vi "HFRR ADV v018 new software.vi"() -> ()   [LabVIEW 2025] (continued)
          tunnel: w2021 -> [_ w2088 _ _]
          frame #0 {
            w2037 = "  " ("String 6")
            n2014 = local write "OPEN"(FALSE ("open")) -> ()
            n2015 = local read "string1 2"() -> (w2025:string)
            n2016 = local read "string1 3"() -> (w2024:string)
            n2017 = local read "string1 4"() -> (w2023:string)
            n2018 = property on="OPEN" class="Bool (strict)"("Visible"=FALSE) -> ()  [unwired: 2 in, 2 out]
            n2019 = local write "String 6"(w2037) -> ()
            n2020 = local write "String 7"(w2037) -> ()
            n2021 = local write "String 8"(w2037) -> ()
            n2022 = local write "String 12"(w2037) -> ()
            n2023 = local read "OK Button 16"() -> (w2022:bool)
            n2024 = String To Path(string=w2025) -> (path=w2033:path)
            n2025 = String To Path(string=w2024) -> (path=w2032:path)
            n2026 = String To Path(string=w2023) -> (path=w2031:path)
            n2027 = case shown="True" w2022 {
              tunnel: [w2038 w2039] -> w2026
              frame False {
                n2028 = local read "string1"() -> (w2038:string)
              }
              frame True {
                n2029 = local read "String Indicator 4"() -> (w2039:string)
              }
            }
            n2030 = Open/Create/Replace File "Open File"(file path (use dialog)=w2033) -> (refnum out=w2029:refnum<file>)  [unwired: 5 in, 2 out]
            n2031 = Open/Create/Replace File "Open File"(file path (use dialog)=w2032) -> (refnum out=w2028:refnum<file>)  [unwired: 5 in, 2 out]
            n2032 = Open/Create/Replace File "Open File"(file path (use dialog)=w2031) -> (refnum out=w2027:refnum<file>)  [unwired: 5 in, 2 out]
            n2033 = while {
              tunnel: w2029 -> [w2051]
              i -> [w2047]
              stop <- w2046 continue-if-true
              (unwired) TRUE ("line mode (F)")
              n2034 = Read from Text File "Read File"(file (use dialog)=w2051) -> (text=w2048:string)  [unwired: 3 in, 3 out]
              n2035 = local write "Numeric 11"(w2047) -> ()
              n2036 = String Length(string=w2048) -> (length=w2050:i32)
              n2037 = Greater?(x=w2050, y=1) -> (0:w2046:bool)
            }
            n2038 = while {
              tunnel: w2028 -> [w2057]
              i -> [w2053]
              stop <- w2052 continue-if-true
              (unwired) TRUE ("line mode (F)")
              n2039 = Read from Text File "Read File"(file (use dialog)=w2057) -> (text=w2054:string)  [unwired: 3 in, 3 out]
              n2040 = local write "Numeric 12"(w2053) -> ()
              n2041 = String Length(string=w2054) -> (length=w2056:i32)
              n2042 = Greater?(x=w2056, y=1) -> (0:w2052:bool)
            }
            n2043 = while {
              tunnel: w2027 -> [w2063]
              i -> [w2059]
              stop <- w2058 continue-if-true
              (unwired) TRUE ("line mode (F)")
              n2044 = Read from Text File "Read File"(file (use dialog)=w2063) -> (text=w2060:string)  [unwired: 3 in, 3 out]
              n2045 = local write "Numeric 13"(w2059) -> ()
              n2046 = String Length(string=w2060) -> (length=w2062:i32)
              n2047 = Greater?(x=w2062, y=1) -> (0:w2058:bool)
            }
            n2048 = String To Path(string=w2026) -> (path=w2034:path)
            n2049 = Open/Create/Replace File "Open File"(file path (use dialog)=w2034) -> (refnum out=w2030:refnum<file>)  [unwired: 5 in, 2 out]
            n2050 = while {
              tunnel: w2030 -> [w2045]
              i -> [w2041]
              stop <- w2040 continue-if-true
              (unwired) TRUE ("line mode (F)")
              n2051 = Read from Text File "Read File"(file (use dialog)=w2045) -> (text=w2042:string)  [unwired: 3 in, 3 out]
              n2052 = local write "Numeric 8"(w2041) -> ()
              n2053 = String Length(string=w2042) -> (length=w2044:i32)
              n2054 = Greater?(x=w2044, y=1) -> (0:w2040:bool)
            }
          }
          frame #1 {
            w2215 = FALSE ("ACTUAL   MERGE")
            # "Sample Temp"
            # "ECR"
            # "COF"
            # "Time\nCOF\nFF\nTemp"
            n2055 = case shown="True" w2088 {
              tunnel: [w2235 w2236] -> w2089
              frame False {
                n2056 = local read "string1"() -> (w2235:string)
              }
              frame True {
                n2057 = local read "String Indicator 4"() -> (w2236:string)
              }
            }
            n2058 = local read "string1 3"() -> (w2133:string)
            n2059 = String To Path(string=w2089) -> (path=w2220:path)
            n2060 = String To Path(string=w2133) -> (path=w2231:path)
            n2061 = local read "Numeric 12"() -> (w2217:i32)
            n2062 = local read "Numeric 8"() -> (w2219:i32)
            n2063 = local read "string1 2"() -> (w2134:string)
            n2064 = local read "string1 4"() -> (w2132:string)
            n2065 = Open/Create/Replace File "Open File"(file path (use dialog)=w2220) -> (refnum out=w2234:refnum<file>, error out=w2233:errorcluster)  [unwired: 5 in, 1 out]
            n2066 = Open/Create/Replace File "Open File"(file path (use dialog)=w2231) -> (refnum out=w2227:refnum<file>, error out=w2228:errorcluster)  [unwired: 5 in, 1 out]
            n2067 = for {
              N: w2219 -> [_]
              tunnel: w2234 -> [w2382]
              tunnel: w2233 -> [w2381]
              tunnel: [w2371] -> w2146 mode=indexing
              tunnel: [w2369] -> w2203 mode=indexing
              tunnel: [w2370] -> w2198 mode=indexing
              tunnel: w2215 -> [_]
              tunnel: [w2363] -> w2200 mode=indexing
              tunnel: [w2359] -> w2169 mode=indexing
              tunnel: [w2355] -> w2144 mode=indexing
              tunnel: [w2351] -> w2125 mode=indexing
              tunnel: [w2346] -> w2085 mode=indexing
              (unwired) TRUE ("line mode (F)")
              # "freq"
              # "Stroke"
              # "Time"
              # "CoF"
              # "Humidity"
              # "Temp"
              # "Air Temp"
              # "ECR"
              n2068 = Read from Text File "Read File"(file (use dialog)=w2382, error in=w2381) -> (text=w2347:string)  [unwired: 2 in, 3 out]
              n2069 = local write "String 6"(w2347) -> ()
              n2070 = String Subset(string=w2347, offset (0)=0, length (rest)=14 ("length (rest)")) -> (substring=w2375:string)
              n2071 = String Subset(string=w2347, offset (0)=35, length (rest)=9 ("length (rest)")) -> (substring=w2372:string)
              n2072 = String Subset(string=w2347, offset (0)=15, length (rest)=9 ("length (rest)")) -> (substring=w2378:string)
              n2073 = Fract/Exp String To Number(string=w2375) -> (number=w2371:dbl)  [unwired: 3 in, 1 out]
              n2074 = Fract/Exp String To Number(string=w2372) -> (number=w2370:dbl)  [unwired: 3 in, 1 out]
              n2075 = Fract/Exp String To Number(string=w2378) -> (number=w2369:dbl)  [unwired: 3 in, 1 out]
              n2076 = String Subset(string=w2347, offset (0)=85, length (rest)=9 ("length (rest)")) -> (substring=w2348:string)
              n2077 = String Subset(string=w2347, offset (0)=25, length (rest)=9 ("length (rest)")) -> (substring=w2354:string)
              n2078 = String Subset(string=w2347, offset (0)=55, length (rest)=9 ("length (rest)")) -> (substring=w2356:string)
              n2079 = String Subset(string=w2347, offset (0)=45, length (rest)=9 ("length (rest)")) -> (substring=w2362:string)
              n2080 = String Subset(string=w2347, offset (0)=65, length (rest)=9 ("length (rest)")) -> (substring=w2368:string)
              n2081 = Fract/Exp String To Number(string=w2354) -> (number=w2351:dbl)  [unwired: 3 in, 1 out]
              n2082 = Fract/Exp String To Number(string=w2348) -> (number=w2346:dbl)  [unwired: 3 in, 1 out]
              n2083 = Fract/Exp String To Number(string=w2356) -> (number=w2355:dbl)  [unwired: 3 in, 1 out]
              n2084 = Fract/Exp String To Number(string=w2362) -> (number=w2359:dbl)  [unwired: 3 in, 1 out]
              n2085 = Fract/Exp String To Number(string=w2368) -> (number=w2365:dbl)  [unwired: 3 in, 1 out]
              n2086 = Add(x=w2365, y=0.0) -> (x+y=w2363:dbl)
            }
            n2087 = for {
              N: w2217 -> [_]
              tunnel: w2228 -> [w2308]
              tunnel: w2227 -> [w2307]
              tunnel: [w2297] -> w2186 mode=indexing
              tunnel: [w2295] -> w2184 mode=indexing
              tunnel: [w2296] -> w2180 mode=indexing
              tunnel: w2215 -> [_]
              tunnel: [w2289] -> w2182 mode=indexing
              tunnel: [w2285] -> w2164 mode=indexing
              tunnel: [w2281] -> w2140 mode=indexing
              tunnel: [w2278] -> w2121 mode=indexing
              tunnel: [w2274] -> w2080 mode=indexing
              (unwired) 9 ("length (rest)")
              (unwired) 9 ("length (rest)")
              (unwired) TRUE ("line mode (F)")
              n2088 = Read from Text File "Read File"(file (use dialog)=w2307, error in=w2308) -> (text=w2275:string)  [unwired: 2 in, 3 out]
              n2089 = local write "String 8"(w2275) -> ()
              n2090 = String Subset(string=w2275, offset (0)=85) -> (substring=w2277:string)  [unwired: 1 in]
              n2091 = String Subset(string=w2275, offset (0)=35, length (rest)=9 ("length (rest)")) -> (substring=w2298:string)
              n2092 = String Subset(string=w2275, offset (0)=55, length (rest)=9 ("length (rest)")) -> (substring=w2283:string)
              n2093 = String Subset(string=w2275, offset (0)=25) -> (substring=w2279:string)  [unwired: 1 in]
              n2094 = String Subset(string=w2275, offset (0)=15, length (rest)=9 ("length (rest)")) -> (substring=w2304:string)
              n2095 = String Subset(string=w2275, offset (0)=0, length (rest)=14 ("length (rest)")) -> (substring=w2301:string)
              n2096 = String Subset(string=w2275, offset (0)=45, length (rest)=9 ("length (rest)")) -> (substring=w2288:string)
              n2097 = String Subset(string=w2275, offset (0)=65, length (rest)=9 ("length (rest)")) -> (substring=w2294:string)
              n2098 = Fract/Exp String To Number(string=w2277) -> (number=w2274:dbl)  [unwired: 3 in, 1 out]
              n2099 = Fract/Exp String To Number(string=w2298) -> (number=w2296:dbl)  [unwired: 3 in, 1 out]
              n2100 = Fract/Exp String To Number(string=w2283) -> (number=w2281:dbl)  [unwired: 3 in, 1 out]
              n2101 = Fract/Exp String To Number(string=w2279) -> (number=w2278:dbl)  [unwired: 3 in, 1 out]
              n2102 = Fract/Exp String To Number(string=w2304) -> (number=w2295:dbl)  [unwired: 3 in, 1 out]
              n2103 = Fract/Exp String To Number(string=w2301) -> (number=w2297:dbl)  [unwired: 3 in, 1 out]
              n2104 = Fract/Exp String To Number(string=w2288) -> (number=w2285:dbl)  [unwired: 3 in, 1 out]
              n2105 = Fract/Exp String To Number(string=w2294) -> (number=w2291:dbl)  [unwired: 3 in, 1 out]
              n2106 = Add(x=w2291, y=0.0) -> (x+y=w2289:dbl)
            }
            n2107 = String To Path(string=w2134) -> (path=w2232:path)
            n2108 = String To Path(string=w2132) -> (path=w2226:path)
            n2109 = local read "Numeric 11"() -> (w2216:i32)
            n2110 = local read "Numeric 13"() -> (w2218:i32)
            n2111 = Open/Create/Replace File "Open File"(file path (use dialog)=w2232) -> (refnum out=w2230:refnum<file>, error out=w2229:errorcluster)  [unwired: 5 in, 1 out]
            n2112 = Open/Create/Replace File "Open File"(file path (use dialog)=w2226) -> (refnum out=w2225:refnum<file>, error out=w2224:errorcluster)  [unwired: 5 in, 1 out]
            n2113 = for {
              N: w2216 -> [_]
              tunnel: w2230 -> [w2345]
              tunnel: w2229 -> [w2344]
              tunnel: [w2334] -> w2196 mode=indexing
              tunnel: [w2332] -> w2194 mode=indexing
              tunnel: [w2333] -> w2189 mode=indexing
              tunnel: w2215 -> [_]
              tunnel: [w2326] -> w2191 mode=indexing
              tunnel: [w2322] -> w2167 mode=indexing
              tunnel: [w2318] -> w2142 mode=indexing
              tunnel: [w2314] -> w2123 mode=indexing
              tunnel: [w2309] -> w2081 mode=indexing
              (unwired) TRUE ("line mode (F)")
              n2114 = Read from Text File "Read File"(file (use dialog)=w2345, error in=w2344) -> (text=w2310:string)  [unwired: 2 in, 3 out]
              n2115 = local write "String 7"(w2310) -> ()
              n2116 = String Subset(string=w2310, offset (0)=85, length (rest)=9 ("length (rest)")) -> (substring=w2313:string)
              n2117 = String Subset(string=w2310, offset (0)=35, length (rest)=9 ("length (rest)")) -> (substring=w2335:string)
              n2118 = String Subset(string=w2310, offset (0)=55, length (rest)=9 ("length (rest)")) -> (substring=w2321:string)
              n2119 = String Subset(string=w2310, offset (0)=25, length (rest)=9 ("length (rest)")) -> (substring=w2315:string)
              n2120 = String Subset(string=w2310, offset (0)=45, length (rest)=9 ("length (rest)")) -> (substring=w2323:string)
              n2121 = String Subset(string=w2310, offset (0)=0, length (rest)=14 ("length (rest)")) -> (substring=w2338:string)
              n2122 = String Subset(string=w2310, offset (0)=15, length (rest)=9 ("length (rest)")) -> (substring=w2341:string)
              n2123 = String Subset(string=w2310, offset (0)=65, length (rest)=9 ("length (rest)")) -> (substring=w2327:string)
              n2124 = Fract/Exp String To Number(string=w2313) -> (number=w2309:dbl)  [unwired: 3 in, 1 out]
              n2125 = Fract/Exp String To Number(string=w2335) -> (number=w2333:dbl)  [unwired: 3 in, 1 out]
              n2126 = Fract/Exp String To Number(string=w2321) -> (number=w2318:dbl)  [unwired: 3 in, 1 out]
              n2127 = Fract/Exp String To Number(string=w2315) -> (number=w2314:dbl)  [unwired: 3 in, 1 out]
              n2128 = Fract/Exp String To Number(string=w2323) -> (number=w2322:dbl)  [unwired: 3 in, 1 out]
              n2129 = Fract/Exp String To Number(string=w2338) -> (number=w2334:dbl)  [unwired: 3 in, 1 out]
              n2130 = Fract/Exp String To Number(string=w2341) -> (number=w2332:dbl)  [unwired: 3 in, 1 out]
              n2131 = Fract/Exp String To Number(string=w2327) -> (number=w2330:dbl)  [unwired: 3 in, 1 out]
              n2132 = Add(x=w2330, y=0.0) -> (x+y=w2326:dbl)
            }
            n2133 = for {
              N: w2218 -> [_]
              tunnel: w2225 -> [w2273]
              tunnel: w2224 -> [w2272]
              tunnel: [w2262] -> w2178 mode=indexing
              tunnel: [w2261] -> w2171 mode=indexing
              tunnel: w2215 -> [_]
              tunnel: [w2250] -> w2176 mode=indexing
              tunnel: [w2255] -> w2173 mode=indexing
              tunnel: [w2251] -> w2163 mode=indexing
              tunnel: [w2246] -> w2138 mode=indexing
              tunnel: [w2242] -> w2119 mode=indexing
              tunnel: [w2237] -> w2079 mode=indexing
              (unwired) 1.0 ("x")
              (unwired) TRUE ("line mode (F)")
              n2134 = Read from Text File "Read File"(file (use dialog)=w2273, error in=w2272) -> (text=w2238:string)  [unwired: 2 in, 3 out]
              n2135 = local write "String 12"(w2238) -> ()
              n2136 = String Subset(string=w2238, offset (0)=85, length (rest)=9 ("length (rest)")) -> (substring=w2240:string)
              n2137 = String Subset(string=w2238, offset (0)=35, length (rest)=9 ("length (rest)")) -> (substring=w2263:string)
              n2138 = String Subset(string=w2238, offset (0)=55, length (rest)=9 ("length (rest)")) -> (substring=w2248:string)
              n2139 = String Subset(string=w2238, offset (0)=25, length (rest)=9 ("length (rest)")) -> (substring=w2244:string)
              n2140 = String Subset(string=w2238, offset (0)=45, length (rest)=9 ("length (rest)")) -> (substring=w2253:string)
              n2141 = String Subset(string=w2238, offset (0)=15, length (rest)=9 ("length (rest)")) -> (substring=w2269:string)
              n2142 = String Subset(string=w2238, offset (0)=0, length (rest)=14 ("length (rest)")) -> (substring=w2266:string)
              n2143 = String Subset(string=w2238, offset (0)=65, length (rest)=9 ("length (rest)")) -> (substring=w2256:string)
              n2144 = Fract/Exp String To Number(string=w2240) -> (number=w2237:dbl)  [unwired: 3 in, 1 out]
              n2145 = Fract/Exp String To Number(string=w2263) -> (number=w2261:dbl)  [unwired: 3 in, 1 out]
              n2146 = Fract/Exp String To Number(string=w2248) -> (number=w2246:dbl)  [unwired: 3 in, 1 out]
              n2147 = Fract/Exp String To Number(string=w2244) -> (number=w2242:dbl)  [unwired: 3 in, 1 out]
              n2148 = Fract/Exp String To Number(string=w2253) -> (number=w2251:dbl)  [unwired: 3 in, 1 out]
              n2149 = Fract/Exp String To Number(string=w2269) -> (number=w2250:dbl)  [unwired: 3 in, 1 out]
              n2150 = Fract/Exp String To Number(string=w2266) -> (number=w2262:dbl)  [unwired: 3 in, 1 out]
              n2151 = Fract/Exp String To Number(string=w2256) -> (number=w2259:dbl)  [unwired: 3 in, 1 out]
              n2152 = Add(x=w2259, y=0.0) -> (x+y=w2255:dbl)
            }
            n2153 = Delete From Array(array=w2121, index=0) -> (array with subset deleted=w2094:dbl[])  [unwired: 1 in, 1 out]
            n2154 = Delete From Array(array=w2184, index=0) -> (array with subset deleted=w2157:dbl[])  [unwired: 1 in, 1 out]
            n2155 = Delete From Array(array=w2164, index=0) -> (array with subset deleted=w2152:dbl[])  [unwired: 1 in, 1 out]
            n2156 = Delete From Array(array=w2182, index=0) -> (array with subset deleted=w2183:dbl[])  [unwired: 1 in, 1 out]
            n2157 = call-poly <vilib>:"Mean.vi"("X"=w2094) -> ("mean"=→"КОФ2 4":dbl)  [unwired: 1 out]
            n2158 = call-poly <vilib>:"Mean.vi"("X"=w2157) -> ("mean"=→"КОФ3":dbl)  [unwired: 1 out]
            n2159 = call-poly <vilib>:"Mean.vi"("X"=w2152) -> ("mean"=→"CP3":dbl)  [unwired: 1 out]
            n2160 = Delete From Array(array=w2146, index=0) -> (array with subset deleted=w2073:dbl[])  [unwired: 1 in, 1 out]
            n2161 = Delete From Array(array=w2085, index=0) -> (array with subset deleted=w2072:dbl[])  [unwired: 1 in, 1 out]
            n2162 = Delete From Array(array=w2125, index=0) -> (array with subset deleted=w2096:dbl[])  [unwired: 1 in, 1 out]
            n2163 = Delete From Array(array=w2203, index=0) -> (array with subset deleted=w2158:dbl[])  [unwired: 1 in, 1 out]
            n2164 = Delete From Array(array=w2169, index=0) -> (array with subset deleted=w2154:dbl[])  [unwired: 1 in, 1 out]
            "array w/ subset deleted" <- w2154
            n2165 = Delete From Array(array=w2200, index=0) -> (array with subset deleted=w2201:dbl[])  [unwired: 1 in, 1 out]
            n2166 = call-poly <vilib>:"Mean.vi"("X"=w2096) -> ("mean"=→"КОФ2 2":dbl)  [unwired: 1 out]
            n2167 = call-poly <vilib>:"Mean.vi"("X"=w2158) -> ("mean"=→"КОФ1":dbl)  [unwired: 1 out]
            n2168 = Bundle "Bundle"(w2073, w2072) -> (w2078:cluster{dbl[], dbl[]})  [unwired: 1 in]
            n2169 = Bundle "Bundle"(w2073, w2201) -> (w2065:cluster{dbl[], dbl[]})  [unwired: 1 in]
            n2170 = Delete From Array(array=w2080, index=0) -> (array with subset deleted=w2068:dbl[])  [unwired: 1 in, 1 out]
            n2171 = Delete From Array(array=w2081, index=0) -> (array with subset deleted=w2070:dbl[])  [unwired: 1 in, 1 out]
            n2172 = Delete From Array(array=w2191, index=0) -> (array with subset deleted=w2192:dbl[])  [unwired: 1 in, 1 out]
            n2173 = Delete From Array(array=w2079, index=0) -> (array with subset deleted=w2066:dbl[])  [unwired: 1 in, 1 out]
            n2174 = Delete From Array(array=w2173, index=0) -> (array with subset deleted=w2174:dbl[])  [unwired: 1 in, 1 out]
            n2175 = Delete From Array(array=w2198, index=0) -> (array with subset deleted=w2104:dbl[])  [unwired: 1 in, 1 out]
            n2176 = Delete From Array(array=w2144, index=0) -> (array with subset deleted=w2100:dbl[])  [unwired: 1 in, 1 out]
            n2177 = Delete From Array(array=w2180, index=0) -> (array with subset deleted=w2102:dbl[])  [unwired: 1 in, 1 out]
            n2178 = Delete From Array(array=w2140, index=0) -> (array with subset deleted=w2098:dbl[])  [unwired: 1 in, 1 out]
            n2179 = Delete From Array(array=w2189, index=0) -> (array with subset deleted=w2103:dbl[])  [unwired: 1 in, 1 out]
            n2180 = Delete From Array(array=w2142, index=0) -> (array with subset deleted=w2099:dbl[])  [unwired: 1 in, 1 out]
            n2181 = Delete From Array(array=w2123, index=0) -> (array with subset deleted=w2095:dbl[])  [unwired: 1 in, 1 out]
            n2182 = Delete From Array(array=w2167, index=0) -> (array with subset deleted=w2153:dbl[])  [unwired: 1 in, 1 out]
            n2183 = Delete From Array(array=w2194, index=0) -> (array with subset deleted=w2155:dbl[])  [unwired: 1 in, 1 out]
            n2184 = Delete From Array(array=w2171, index=0) -> (array with subset deleted=w2101:dbl[])  [unwired: 1 in, 1 out]
            n2185 = Delete From Array(array=w2138, index=0) -> (array with subset deleted=w2097:dbl[])  [unwired: 1 in, 1 out]
            n2186 = Delete From Array(array=w2119, index=0) -> (array with subset deleted=w2093:dbl[])  [unwired: 1 in, 1 out]
            n2187 = Delete From Array(array=w2163, index=0) -> (array with subset deleted=w2151:dbl[])  [unwired: 1 in, 1 out]
            n2188 = Delete From Array(array=w2176, index=0) -> (array with subset deleted=w2156:dbl[])  [unwired: 1 in, 1 out]
            n2189 = Delete From Array(array=w2186, index=0) -> (array with subset deleted=w2069:dbl[])  [unwired: 1 in, 1 out]
            n2190 = Delete From Array(array=w2196, index=0) -> (array with subset deleted=w2071:dbl[])  [unwired: 1 in, 1 out]
            n2191 = Delete From Array(array=w2178, index=0) -> (array with subset deleted=w2067:dbl[])  [unwired: 1 in, 1 out]
            n2192 = Bundle "Bundle"(w2073, w2104) -> (w2091:cluster{dbl[], dbl[]})  [unwired: 1 in]
            n2193 = Bundle "Bundle"(w2073, w2158) -> (w2092:cluster{dbl[], dbl[]})  [unwired: 1 in]
            n2194 = Bundle "Bundle"(w2104, w2100) -> (w2106:cluster{dbl[], dbl[]})  [unwired: 1 in]
            n2195 = Bundle "Bundle"(w2069, w2068) -> (w2076:cluster{dbl[], dbl[]})  [unwired: 1 in]
            n2196 = Bundle "Bundle"(w2102, w2098) -> (w2108:cluster{dbl[], dbl[]})  [unwired: 1 in]
            n2197 = Bundle "Bundle"(w2069, w2102) -> (w2212:cluster{dbl[], dbl[]})  [unwired: 1 in]
            n2198 = Bundle "Bundle"(w2069, w2098) -> (w2136:cluster{dbl[], dbl[]})  [unwired: 1 in]
            n2199 = Bundle "Bundle"(w2069, w2157) -> (w2222:cluster{dbl[], dbl[]})  [unwired: 1 in]
            n2200 = Bundle "Bundle"(w2069, w2152) -> (w2160:cluster{dbl[], dbl[]})  [unwired: 1 in]
            n2201 = Bundle "Bundle"(w2069, w2183) -> (w2207:cluster{dbl[], dbl[]})  [unwired: 1 in]
            n2202 = Bundle "Bundle"(w2103, w2099) -> (w2107:cluster{dbl[], dbl[]})  [unwired: 1 in]
            n2203 = Bundle "Bundle"(w2071, w2070) -> (w2077:cluster{dbl[], dbl[]})  [unwired: 1 in]
            n2204 = Bundle "Bundle"(w2071, w2103) -> (w2214:cluster{dbl[], dbl[]})  [unwired: 1 in]
            n2205 = Bundle "Bundle"(w2071, w2099) -> (w2137:cluster{dbl[], dbl[]})  [unwired: 1 in]
            n2206 = Bundle "Bundle"(w2071, w2153) -> (w2161:cluster{dbl[], dbl[]})  [unwired: 1 in]
            n2207 = Bundle "Bundle"(w2071, w2155) -> (w2223:cluster{dbl[], dbl[]})  [unwired: 1 in]
            n2208 = Bundle "Bundle"(w2071, w2192) -> (w2205:cluster{dbl[], dbl[]})  [unwired: 1 in]
            n2209 = Bundle "Bundle"(w2101, w2097) -> (w2109:cluster{dbl[], dbl[]})  [unwired: 1 in]
            n2210 = Bundle "Bundle"(w2067, w2066) -> (w2075:cluster{dbl[], dbl[]})  [unwired: 1 in]
            n2211 = Bundle "Bundle"(w2067, w2101) -> (w2213:cluster{dbl[], dbl[]})  [unwired: 1 in]
            n2212 = Bundle "Bundle"(w2067, w2097) -> (w2135:cluster{dbl[], dbl[]})  [unwired: 1 in]
            n2213 = Bundle "Bundle"(w2067, w2151) -> (w2159:cluster{dbl[], dbl[]})  [unwired: 1 in]
            n2214 = Bundle "Bundle"(w2067, w2156) -> (w2221:cluster{dbl[], dbl[]})  [unwired: 1 in]
            n2215 = Bundle "Bundle"(w2067, w2174) -> (w2206:cluster{dbl[], dbl[]})  [unwired: 1 in]
            n2216 = call-poly <vilib>:"Mean.vi"("X"=w2154) -> ("mean"=→"CP1":dbl)  [unwired: 1 out]
            n2217 = call-poly <vilib>:"Mean.vi"("X"=w2095) -> ("mean"=→"КОФ2 3":dbl)  [unwired: 1 out]
            n2218 = call-poly <vilib>:"Mean.vi"("X"=w2153) -> ("mean"=→"CP2":dbl)  [unwired: 1 out]
            n2219 = call-poly <vilib>:"Mean.vi"("X"=w2155) -> ("mean"=→"КОФ2":dbl)  [unwired: 1 out]
            n2220 = call-poly <vilib>:"Mean.vi"("X"=w2093) -> ("mean"=→"КОФ2 5":dbl)  [unwired: 1 out]
            n2221 = call-poly <vilib>:"Mean.vi"("X"=w2151) -> ("mean"=→"CP4":dbl)  [unwired: 1 out]
            n2222 = call-poly <vilib>:"Mean.vi"("X"=w2156) -> ("mean"=→"КОФ4":dbl)  [unwired: 1 out]
            n2223 = Bundle "Bundle"(w2073, w2100) -> (w2064:cluster{dbl[], dbl[]})  [unwired: 1 in]
            n2224 = Bundle "Bundle"(w2073, w2154) -> (w2087:cluster{dbl[], dbl[]})  [unwired: 1 in]
            n2225 = Build Array "Build Array"(w2064, w2087) -> (w2090:cluster{dbl[], dbl[]}[])
            "XY Graph 17" <- w2090
            n2226 = Build Array "Build Array"(w2078, w2077, w2076, w2075) -> (→"Frequency ( Hz )":cluster{dbl[], dbl[]}[])
            n2227 = Build Array "Build Array"(w2106, w2107, w2108, w2109) -> (→"Air Temp ( °C ) vs Humidity ( % RH )":cluster{dbl[], dbl[]}[])
            n2228 = Build Array "Build Array"(w2091, w2214, w2212, w2213) -> (→"Air Temperature  ( °C )":cluster{dbl[], dbl[]}[])
            n2229 = Build Array "Build Array"(w2064, w2137, w2136, w2135) -> (→"Humidity ( %RH )":cluster{dbl[], dbl[]}[])
            n2230 = Build Array "Build Array"(w2092, w2223, w2222, w2221) -> (→"Coefficient Of Friction":cluster{dbl[], dbl[]}[])
            n2231 = Build Array "Build Array"(w2087, w2161, w2160, w2159) -> (→"Sample Temperature ( °C )":cluster{dbl[], dbl[]}[])
            n2232 = Build Array "Build Array"(w2065, w2205, w2207, w2206) -> (→"XY Graph 13":cluster{dbl[], dbl[]}[])
            n2233 = Bundle "Bundle"(w2073, w2096) -> (w2118:cluster{dbl[], dbl[]})  [unwired: 1 in]
            n2234 = Bundle "Bundle"(w2069, w2094) -> (w2116:cluster{dbl[], dbl[]})  [unwired: 1 in]
            n2235 = Bundle "Bundle"(w2071, w2095) -> (w2117:cluster{dbl[], dbl[]})  [unwired: 1 in]
            n2236 = Bundle "Bundle"(w2067, w2093) -> (w2115:cluster{dbl[], dbl[]})  [unwired: 1 in]
            n2237 = Build Array "Build Array"(w2118, w2117, w2116, w2115) -> (→"Stroke ( mm )":cluster{dbl[], dbl[]}[])
            n2238 = local write "XY Graph 16"(w2090) -> ()
          }
          frame #2 {
          }
          frame #3 {
            n2239 = local write "Numeric 8"(0 ("Numeric 8")) -> ()
            n2240 = local write "Numeric 11"(0 ("Numeric 11")) -> ()
            n2241 = local write "Numeric 12"(0 ("Numeric 12")) -> ()
            n2242 = local write "Numeric 13"(0 ("Numeric 13")) -> ()
            n2243 = property on="OPEN" class="Bool (strict)"("Visible"=TRUE) -> ()  [unwired: 2 in, 2 out]
            n2244 = local read "String Control 2"() -> (w2390:string)
            n2245 = local read "String Control 4"() -> (w2389:string)
            n2246 = local read "String Control 6"() -> (w2388:string)
            n2247 = local read "String Control 8"() -> (w2387:string)
            n2248 = Match Pattern(string=w2390, regular expression="Samples / cycle :- ") -> (after substring=w2404:string)  [unwired: 1 in, 3 out]
            n2249 = Match Pattern(string=w2390, regular expression="Frequency :- ") -> (after substring=w2423:string)  [unwired: 1 in, 3 out]
            n2250 = Match Pattern(string=w2389, regular expression="Samples / cycle :- ") -> (after substring=w2400:string)  [unwired: 1 in, 3 out]
            n2251 = Match Pattern(string=w2389, regular expression="Frequency :- ") -> (after substring=w2418:string)  [unwired: 1 in, 3 out]
            n2252 = Match Pattern(string=w2388, regular expression="Samples / cycle :- ") -> (after substring=w2396:string)  [unwired: 1 in, 3 out]
            n2253 = Match Pattern(string=w2388, regular expression="Frequency :- ") -> (after substring=w2413:string)  [unwired: 1 in, 3 out]
            n2254 = Match Pattern(string=w2387, regular expression="Samples / cycle :- ") -> (after substring=w2392:string)  [unwired: 1 in, 3 out]
            n2255 = Match Pattern(string=w2387, regular expression="Frequency :- ") -> (after substring=w2408:string)  [unwired: 1 in, 3 out]
            n2256 = String Subset(string=w2404, length (rest)=6 ("length (rest)")) -> (substring=w2406:string)  [unwired: 1 in]
            n2257 = String Subset(string=w2423, length (rest)=9 ("length (rest)")) -> (substring=w2425:string)  [unwired: 1 in]
            n2258 = String Subset(string=w2400, length (rest)=6 ("length (rest)")) -> (substring=w2402:string)  [unwired: 1 in]
            n2259 = String Subset(string=w2418, length (rest)=9 ("length (rest)")) -> (substring=w2420:string)  [unwired: 1 in]
            n2260 = String Subset(string=w2396, length (rest)=6 ("length (rest)")) -> (substring=w2398:string)  [unwired: 1 in]
            n2261 = String Subset(string=w2413, length (rest)=9 ("length (rest)")) -> (substring=w2415:string)  [unwired: 1 in]
            n2262 = String Subset(string=w2392, length (rest)=6 ("length (rest)")) -> (substring=w2394:string)  [unwired: 1 in]
            n2263 = String Subset(string=w2408, length (rest)=9 ("length (rest)")) -> (substring=w2410:string)  [unwired: 1 in]
            n2264 = Fract/Exp String To Number(string=w2406) -> (number=w2386:dbl)  [unwired: 3 in, 1 out]
            n2265 = Fract/Exp String To Number(string=w2425) -> (number=w2426:dbl)  [unwired: 3 in, 1 out]
            n2266 = Fract/Exp String To Number(string=w2402) -> (number=w2385:dbl)  [unwired: 3 in, 1 out]
            n2267 = Fract/Exp String To Number(string=w2420) -> (number=w2421:dbl)  [unwired: 3 in, 1 out]
            n2268 = Fract/Exp String To Number(string=w2398) -> (number=w2384:dbl)  [unwired: 3 in, 1 out]
            n2269 = Fract/Exp String To Number(string=w2415) -> (number=w2416:dbl)  [unwired: 3 in, 1 out]
            n2270 = Fract/Exp String To Number(string=w2394) -> (number=w2383:dbl)  [unwired: 3 in, 1 out]
            n2271 = Fract/Exp String To Number(string=w2410) -> (number=w2411:dbl)  [unwired: 3 in, 1 out]
            n2272 = local write "sample1"(w2386) -> ()
            n2273 = local write "freq1"(w2426) -> ()
            n2274 = local write "sample2"(w2385) -> ()
            n2275 = local write "freq2"(w2421) -> ()
            n2276 = local write "sample3"(w2384) -> ()
            n2277 = local write "freq3"(w2416) -> ()
            n2278 = local write "sample4"(w2383) -> ()
            n2279 = local write "freq 4"(w2411) -> ()
          }
        }
      }
    }
    n2280 = case shown="True" w1875 {
      selector: w1875 -> [_ w2003]
      frame False {
      }
      frame True {
        n2281 = Not(x=w2003) -> (.not. x?=w1999:bool)
        n2282 = local write "service 3"(w1999) -> ()
        n2283 = local write "OPEN 6"(w1999) -> ()
        n2284 = call <vilib>:"System Exec.vi"("wait until completion? (T)"=TRUE, "command line"="C:\\LAB-IQ\\Scar View.exe") -> ("error out"=→"error out 5":errorcluster)  [unwired: 6 in, 3 out]
      }
    }
    n2285 = case shown="\"Acquire\", Default" w1886 {
      frame "Acquire", Default {
        w2899 = 0.2 ("y")
        w2904 = 1.0 ("y")
        w2905 = 0.8 ("y")
        # "Elapsed time\ncof\nstroke\nAir temp\nTemp\nHumidity"
        n2286 = disable-structure shown="Disabled" {
          frame Disabled {
            n2287 = local read "Flag"() -> (w2922:dbl)
            n2288 = local read "RUN"() -> (w2919:bool)
            n2289 = Not(x=w2919) -> (.not. x?=w2918:bool)
            n2290 = Equal?(x=w2922, y=10.0) -> (x = y?=w2920:bool)
            n2291 = And(x=w2920, y=w2918) -> (x .and. y?=w2917:bool)
            n2292 = case shown="True" w2917 {
              frame False {
              }
              frame True {
                w2923 = FALSE ("Heater Button")
                n2293 = local write "Humidity"(w2923) -> ()
                n2294 = local write "Heater Button"(w2923) -> ()
              }
            }
          }
          frame Enabled {
          }
        }
        n2295 = disable-structure shown="Disabled" {
          frame Disabled {
            n2296 = case shown="True" {
              selector: _ -> [_ _]
              frame False {
              }
              frame True {
                w3014 = TRUE ("Heater")
                n2297 = local write "Humidity"(w3014) -> ()
                n2298 = local write "Heater Button"(w3014) -> ()
                n2299 = local read "TEST STANDARD"() -> (w3017:T3)
                n2300 = local read "TEST STANDARD"() -> (w3012:T3)
                n2301 = Equal?(x=w3017, y=enum16{"ASTM D6079", "ISO 12156", "Custom"}."ISO 12156" ("Test Standard")) -> (x = y?=w3015:bool)
                n2302 = Equal?(x=w3012, y=enum16{"ASTM D6079", "ISO 12156", "Custom"}."ASTM D6079" ("Test Standard")) -> (x = y?=w3011:bool)
                n2303 = case shown="True" w3015 {
                  frame False {
                  }
                  frame True {
                    n2304 = local write "Heater"(TRUE ("Heater")) -> ()
                    n2305 = local write "airtempflg"(FALSE ("airtempflg")) -> ()
                  }
                }
                n2306 = case shown="True" w3011 {
                  frame False {
                  }
                  frame True {
                    n2307 = local write "Heater"(FALSE ("Heater")) -> ()
                    n2308 = local write "airtempflg"(TRUE ("airtempflg")) -> ()
                  }
                }
              }
            }
          }
          frame Enabled {
          }
        }
        n2309 = stacked-sequence {
          frame #0 {
            n2310 = case shown="True" "RST FF" {
              frame False {
              }
              frame True {
                w3080 = 0.0 ("X Scale.Range:Maximum")
                n2311 = property on="Frictional Force ( N )" class="WFChart (strict)"("XScale.Maximum"=600.0 ("X Scale.Range:Maximum"), "XScale.Minimum"=w3080, "YScale.Maximum"=10.0 ("Y Scale.Range:Maximum"), "YScale.Minimum"=w3080) -> ()  [unwired: 2 in, 2 out]
              }
            }
          }
          frame #1 {
            n2312 = case shown="True" "RST TEMP" {
              frame False {
              }
              frame True {
                n2313 = property on="Temperature ( Deg C )" class="WFChart (strict)"("XScale.Minimum"=0.0 ("X Scale.Range:Minimum"), "XScale.Maximum"=600.0 ("X Scale.Range:Maximum"), "YScale.Minimum"=0.0 ("Y Scale.Range:Minimum"), "YScale.Maximum"=100.0 ("Y Scale.Range:Maximum")) -> ()  [unwired: 2 in, 2 out]
              }
            }
          }
          frame #2 {
            n2314 = case shown="True" "RSTCOF" {
              frame False {
              }
              frame True {
                n2315 = property on="Coefficient of Friction" class="WFChart (strict)"("XScale.Minimum"=0.0 ("X Scale.Range:Minimum"), "XScale.Maximum"=600.0 ("X Scale.Range:Maximum"), "YScale.Maximum"=1.0 ("X Scale.Range:Minimum"), "YScale.Minimum"=0.0 ("X Scale.Range:Minimum")) -> ()  [unwired: 2 in, 2 out]
              }
            }
          }
          frame #3 {
            n2316 = case shown="True" "RSTCOF 2" {
              frame False {
              }
              frame True {
                (unwired) 100.0 ("Y Scale.Range:Maximum")
                (unwired) 0.0 ("Y Scale.Range:Minimum")
                (unwired) 600.0 ("X Scale.Range:Maximum")
                (unwired) 0.0 ("X Scale.Range:Minimum")
              }
            }
          }
          frame #4 {
            n2317 = case shown="True" "RSTCOF 3" {
              frame False {
              }
              frame True {
                n2318 = property on="Electrical Contact Resistance ( % )" class="WFChart (strict)"("XScale.Minimum"=0.0 ("X Scale.Range:Minimum"), "XScale.Maximum"=600.0 ("X Scale.Range:Maximum"), "YScale.Minimum"=0.0 ("Y Scale.Range:Minimum"), "YScale.Maximum"=100.0 ("Y Scale.Range:Maximum")) -> ()  [unwired: 2 in, 2 out]
              }
            }
          }
        }
        n2319 = disable-structure shown="Disabled" {
          frame Disabled {
            n2320 = case shown="True" {
              selector: _ -> [_ _]
              frame False {
              }
              frame True {
                n2321 = local read "zflag 2"() -> (w2981:dbl)
                n2322 = local read "yflag"() -> (w2983:dbl)
                n2323 = Equal?(x=w2983, y=2.0 ("tflag")) -> (x = y?=w2985:bool)
                n2324 = Equal?(x=w2981, y=3.0 ("tflag")) -> (x = y?=w2984:bool)
                n2325 = And(x=w2985, y=w2984) -> (x .and. y?=w2979:bool)
                n2326 = case shown="True" w2979 {
                  frame False {
                  }
                  frame True {
                    w3010 = 0.0 ("zflag")
                    n2327 = local write "zflag"(w3010) -> ()
                    n2328 = local write "zflag 2"(w3010) -> ()
                    n2329 = Delete(path (use dialog)=path "C:/LAB-IQ-NXT/WO 2449 TT.sig" ("file path (dialog if empty)")) -> (deleted path=w3009:path)  [unwired: 4 in, 2 out]
                    n2330 = Delete(path (use dialog)=path "C:/LAB-IQ-NXT/WO 2449 TRH.sig" ("file path (dialog if empty)")) -> (deleted path=w3004:path)  [unwired: 4 in, 2 out]
                    n2331 = local read "SEN.RUN HRS"() -> (w2996:dbl)
                    n2332 = local read "SENSOR TIME"() -> (w2994:dbl)
                    n2333 = call <vilib>:"compatOverwrite.vi"("overwrite (F)"=TRUE) -> ("overwrite?"=w2986:T30)
                    n2334 = call <vilib>:"compatOverwrite.vi"("overwrite (F)"=TRUE) -> ("overwrite?"=w2990:T30)
                    n2335 = local read "Total No. of Tests"() -> (w2997:dbl)
                    n2336 = Add(x=w2994, y=w2996) -> (x+y=w2995:dbl)
                    "SEN.RUN HRS" <- w2995
                    n2337 = Open/Create/Replace File(file path (use dialog)=w3009, operation (0:open)=w2986) -> (refnum out=w2987:refnum<file>, error out=w2988:errorcluster)  [unwired: 4 in, 1 out]
                    n2338 = Open/Create/Replace File(file path (use dialog)=w3004, operation (0:open)=w2990) -> (refnum out=w2991:refnum<file>, error out=w2992:errorcluster)  [unwired: 4 in, 1 out]
                    n2339 = Deny Access(4:w2988, 6:T28."deny none" ("deny mode (2)"), 7:w2987) -> (3:w3008:refnum<file>)  [unwired: 1 out]
                    n2340 = Deny Access(4:w2992, 6:T28."deny none" ("deny mode (2)"), 7:w2991) -> (3:w3000:refnum<file>)  [unwired: 1 out]
                    n2341 = Number To Decimal String(number=w2997) -> (decimal integer string=w3005:string)  [unwired: 1 in]
                    n2342 = Number To Decimal String(number=w2995) -> (decimal integer string=w3001:string)  [unwired: 1 in]
                    n2343 = Write to Binary File(file (use dialog)=w3008, data=w3005, 5:FALSE ("prepend array or string size? (T)")) -> ()  [unwired: 3 in, 3 out]
                    n2344 = Write to Binary File(file (use dialog)=w3000, data=w3001, 5:FALSE ("prepend array or string size? (T)")) -> ()  [unwired: 3 in, 3 out]
                  }
                }
              }
            }
          }
          frame Enabled {
          }
        }
        n2345 = local read "RUN"() -> (w2908:bool)
        n2346 = local read "run replace"() -> (w2912:bool)
        n2347 = local read "run replace"() -> (w2911:bool)
        n2348 = case shown="True" w2908 {
          frame False {
            n2349 = local write "run replace"(FALSE ("run replace")) -> ()
          }
          frame True {
            "run replace" <- TRUE ("run replace")
          }
        }
        n2350 = local read "RUN"() -> (w2916:bool)
        n2351 = local read "Set Temp"() -> (w2878:dbl)
        n2352 = local read "SetTemp"() -> (w2880:dbl)
        n2353 = case shown="False" w2916 {
          tunnel: [FALSE ("TEST RUNNING") TRUE ("TEST RUNNING")] -> w2915
          frame False {
            w3099 = 0.0 ("Flag")
            n2354 = local write "Elapsed time"(0.0 ("elapsedtime")) -> ()
            n2355 = local write "Time Remaining"(w3099) -> ()
            n2356 = local write "Flag"(w3099) -> ()
            n2357 = local write "Remaining Time"(w3099) -> ()
          }
          frame True {
            n2358 = local write "Flag"(10.0 ("Flag")) -> ()
          }
        }
        n2359 = case shown="False" w2912 {
          frame False {
            n2360 = local read "zflag"() -> (→"zflag 2":dbl)
            n2361 = local write "yflag"(2.0 ("tflag")) -> ()
            n2362 = local write "FLAG 4"(0.0 ("FLAG")) -> ()
          }
          frame True {
            n2363 = local write "yflag"(1.0 ("tflag")) -> ()
            n2364 = local write "zflag"(3.0 ("zflag")) -> ()
          }
        }
        n2365 = local read "acq 2"() -> (w2910:bool)
        n2366 = local read "AIR TEMP"() -> (w2873:dbl)
        n2367 = local read "Amb temp"() -> (w2877:dbl)
        n2368 = case shown="True" "Save & Continue" {
          frame False {
          }
          frame True {
            "acq 2" <- TRUE ("acq 2")
          }
        }
        n2369 = local read "Set Rh"() -> (w2879:dbl)
        n2370 = Add(x=w2880, y=w2905) -> (x+y=w2906:dbl)
        n2371 = Subtract(x=w2880, y=w2905) -> (x-y=w2907:dbl)
        n2372 = Add(x=w2878, y=w2899) -> (x+y=w2900:dbl)
        n2373 = Subtract(x=w2878, y=w2899) -> (x-y=w2901:dbl)
        n2374 = And(x=w2910, y=w2911) -> (x .and. y?=w2909:bool)
        n2375 = Greater Or Equal?(x=w2873, y=15.0) -> (x >= y?=w2874:bool)
        "powstat" <- w2874
        n2376 = local read "Humidity ( %RH )"() -> (w2876:dbl)
        n2377 = case shown="True" "Save & Continue" {
          frame False {
          }
          frame True {
            n2378 = while {
              tunnel: "0123456789abcdefghijklmnopqrstuvwxyzABCDEFGHIJKLMNOPQRSTUVWXYZ" ("string 2") -> [w3070]
              shift-right: [w3068] -> w3063
              shift-left: "" -> [w3067]
              i -> [w3077]
              stop <- w3076 stop-if-true
              n2379 = Random Number (0-1)() -> (number: 0 to 1=w3071:dbl)
              n2380 = Multiply(x=w3071, y=62.0) -> (x*y=w3073:dbl)
              n2381 = Decrement(x="Length") -> (x-1=w3066:i16)
              n2382 = To Word Integer(number=w3073) -> (16bit integer=w3074:i16)
              n2383 = String Subset(string=w3070, offset (0)=w3074, length (rest)=1 ("length (rest)")) -> (substring=w3069:string)
              n2384 = Greater Or Equal?(x=w3077, y=w3066) -> (x >= y?=w3076:bool)
              n2385 = Concatenate Strings(w3069, w3067) -> (w3068:string)
            }
            n2386 = local write "UUID"(w3063) -> ()
          }
        }
        n2387 = In Range and Coerce(upper limit=w2906, x=w2877, lower limit=w2907) -> (In Range?=w2896:bool)  [unwired: 1 out]
        n2388 = Add(x=w2879, y=w2904) -> (x+y=w2903:dbl)
        n2389 = Subtract(x=w2879, y=w2904) -> (x-y=w2902:dbl)
        n2390 = local read "TEMP"() -> (w2875:dbl)
        n2391 = case shown="True" "Save & Continue" {
          frame False {
          }
          frame True {
            n2392 = local read "Operator ID"() -> (w3394:string)
            n2393 = local read "FILE"() -> (w3400:string)
            n2394 = String Length(string=w3400) -> (length=w3398:i32)
            n2395 = String Length(string=w3394) -> (length=w3395:i32)
            n2396 = Greater?(x=w3398, y=0) -> (0:w3397:bool)
            n2397 = Greater?(x=w3395, y=0) -> (0:w3393:bool)
            n2398 = And(x=w3397, y=w3393) -> (x .and. y?=w3392:bool)
            n2399 = case shown="True" w3392 {
              frame False {
                n2400 = stacked-sequence {
                  frame #0 {
                    n2401 = One Button Dialog(message="Please Enter a File Name and Operator ID to save data !", button name ("OK")="Ok") -> ()  [unwired: 1 out]
                  }
                  frame #1 {
                    n2402 = local write "Save & Continue"(FALSE ("OK Button")) -> ()
                  }
                }
                n2403 = local write "Save & Continue"(FALSE ("OK Button")) -> ()
              }
              frame True {
                n2404 = stacked-sequence {
                  frame #0 {
                    n2405 = local read "FILE"() -> (w3406:string)
                    n2406 = call "file check.vi"("file name in"=w3406) -> ("file name out"=w3405:string)  [unwired: 9 in, 1 out]
                    n2407 = call <vilib>:"Application Directory.vi"() -> ("Application Directory"=w3416:path)
                    n2408 = Build Path(base path=w3416, name or relative path="data") -> (appended path=w3415:path)
                    n2409 = call <vilib>:"Trim Whitespace.vi"("string"=w3405) -> ("trimmed string"=w3413:string)  [unwired: 1 in]
                    n2410 = call <vilib>:"Trim Whitespace.vi"("string"=w3405) -> ("trimmed string"=w3414:string)  [unwired: 1 in]
                    n2411 = List Folder(path=w3415) -> (folder names=w3411:string[])  [unwired: 3 in, 3 out]
                    n2412 = Match Pattern(string=w3413, regular expression="_(") -> (before substring=w3410:string)  [unwired: 1 in, 3 out]
                    n2413 = for {
                      tunnel: w3411 -> [w3425] mode=indexing
                      tunnel: w3410 -> [w3423]
                      shift-right: [w3421] -> w3408
                      shift-left: bool[] [] -> [w3422]
                      n2414 = Match Pattern(string=w3425, regular expression="_(") -> (before substring=w3424:string)  [unwired: 1 in, 3 out]
                      n2415 = Equal?(x=w3424, y=w3423) -> (x = y?=w3420:bool)
                      n2416 = case shown="True" w3420 {
                        tunnel: w3420 -> [_ w3428]
                        tunnel: w3422 -> [w3427 w3430]
                        tunnel: [w3427 w3429] -> w3421
                        frame False {
                        }
                        frame True {
                          n2417 = Insert Into Array(array=w3430, new element=w3428) -> (w3429:bool[])  [unwired: 1 in]
                        }
                      }
                    }
                    n2418 = Equal?(x=w3411, y=w3410) -> (x = y?=w3419:bool[])
                    n2419 = Or Array Elements(Boolean array=w3419) -> (logical OR=w3418:bool)
                    n2420 = Array Size(array=w3408) -> (size(s)=w3407:i32)
                    n2421 = case shown="True" w3418 {
                      tunnel: w3414 -> [_ w3438]
                      tunnel: w3407 -> [_ w3431]
                      frame False {
                      }
                      frame True {
                        n2422 = Number To Decimal String(number=w3431) -> (decimal integer string=w3434:string)  [unwired: 1 in]
                        n2423 = Search/Split String(string=w3438, search string/char (-)="_(" ("regular expression")) -> (substring before match=w3436:string)  [unwired: 1 in, 2 out]
                        n2424 = Concatenate Strings(w3436, "_(" ("regular expression"), w3434, ")" ("regular expression")) -> (w3432:string)
                        n2425 = local write "FILE"(w3432) -> ()
                      }
                    }
                  }
                  frame #1 {
                    w3440 = 0.0
                    w3453 = cluster{"y":dbl, dbl, "y":dbl}[] [] ("History Data")
                    w3454 = FALSE ("Heater Button")
                    (unwired) ")!" ("string")
                    (unwired) ")" ("string")
                    w3452 = dbl[] [] ("History Data")
                    w3458 = "\r"
                    # "C:\\WinDucom\\Data\\"
                    # "C:\\LAB-IQ-NXT\\data"
                    n2426 = local write "Humidity ( %RH )"(w3440) -> ()
                    n2427 = local write "Frequency ( Hz )"(w3440) -> ()
                    n2428 = local write "Stroke 3"(w3440) -> ()
                    n2429 = local write "speedop"(0.0 ("PIDclk 2")) -> ()
                    n2430 = local write "Set Temp 2"(65.0 ("Set Temp 2")) -> ()
                    n2431 = local write "AIR TEMP"(w3440) -> ()
                    n2432 = local write "clk"(0.0 ("clk")) -> ()
                    n2433 = local write "Stroke 4"(w3440) -> ()
                    n2434 = local write "COF 2"(w3440) -> ()
                    n2435 = local write "TEMP"(w3440) -> ()
                    n2436 = local write "ecr 3"(w3440) -> ()
                    n2437 = local write "FF 3"(w3440) -> ()
                    n2438 = local write "FF 2"(w3440) -> ()
                    n2439 = property on="Humidity ( %RH )" class="WFChart (strict)"("History Data"=w3452) -> ()  [unwired: 2 in, 2 out]
                    n2440 = property on="Coefficient of Friction" class="WFChart (strict)"("History Data"=w3452) -> ()  [unwired: 2 in, 2 out]
                    n2441 = property on="Coefficient of Friction" class="WFChart (strict)"("History Data"=w3452) -> ()  [unwired: 2 in, 2 out]
                    n2442 = property on="Frictional Force ( N )" class="WFChart (strict)"("History Data"=w3452) -> ()  [unwired: 2 in, 2 out]
                    n2443 = property on="Electrical Contact Resistance ( % )" class="WFChart (strict)"("History Data"=w3452) -> ()  [unwired: 2 in, 2 out]
                    n2444 = property on="Electrical Contact Resistance ( % )" class="WFChart (strict)"("History Data"=w3452) -> ()  [unwired: 2 in, 2 out]
                    n2445 = property on="Temperature ( Deg C )" class="WFChart (strict)"("History Data"=w3452) -> ()  [unwired: 2 in, 2 out]
                    n2446 = property on="Frictional Force ( N )" class="WFChart (strict)"("History Data"=w3452) -> ()  [unwired: 2 in, 2 out]
                    n2447 = property on="Coefficient of Friction" class="WFChart (strict)"("History Data"=w3452) -> ()  [unwired: 2 in, 2 out]
                    n2448 = property on="Frictional Force ( N )" class="WFChart (strict)"("History Data"=w3452) -> ()  [unwired: 2 in, 2 out]
                    n2449 = property on="Electrical Contact Resistance ( % )" class="WFChart (strict)"("History Data"=w3452) -> ()  [unwired: 2 in, 2 out]
                    n2450 = property on="Temperature ( Deg C )" class="WFChart (strict)"("History Data"=w3452) -> ()  [unwired: 2 in, 2 out]
                    n2451 = property on="Humidity ( %RH )" class="WFChart (strict)"("History Data"=w3452) -> ()  [unwired: 2 in, 2 out]
                    n2452 = property on="Stroke ( mm )" class="WFChart (strict)"("History Data"=w3453) -> ()  [unwired: 2 in, 2 out]
                    n2453 = property on="Stroke ( mm )" class="WFChart (strict)"("History Data"=w3453) -> ()  [unwired: 2 in, 2 out]
                    n2454 = local write "Humidity"(w3454) -> ()
                    n2455 = local write "Heater Button"(w3454) -> ()
                    n2456 = local read "FILE"() -> (w3448:string)
                    n2457 = disable-structure shown="Enabled" {
                      disable-tunnel: [w3493 _] -> w3439
                      frame Enabled {
                        n2458 = local read "NORMAL LOAD"() -> (w3493:dbl)
                      }
                      frame Disabled {
                      }
                    }
                    n2459 = call "file check.vi"("file name in"=w3448) -> ("error out"=w3451:errorcluster, "file name out"=w3445:string)  [unwired: 9 in]
                    n2460 = call "FILE PATH CREATION.vi"("error in"=w3451, "FILE NAME :"=w3445) -> ("FILE OUT"=w3444:path)  [unwired: 8 in, 1 out]
                    n2461 = Concatenate Strings(w3445, ".dgf" ("Substring")) -> (w3450:string)
                    n2462 = Concatenate Strings(w3445, ".duf" ("Substring")) -> (w3446:string)
                    n2463 = Multiply(x=w3439, y=1.0) -> (x*y=w3472:dbl)
                    n2464 = Build Path(base path=w3444, name or relative path=w3450) -> (appended path=w3443:path)
                    n2465 = Build Path(base path=w3444, name or relative path=w3446) -> (appended path=w3442:path)
                    n2466 = Number To Fractional String(number=w3472, width (-)=i16 5, precision (6)=i16 2) -> (F-format string=w3480:string)  [unwired: 1 in]
                    n2467 = local read "Fuel Discription :"() -> (w3468:string)
                    n2468 = local read "Batch Ref Num :"() -> (w3456:string)
                    n2469 = Get Date/Time String(date format (0)=enum16{"short", "long", "abbreviated"}."short") -> (date string=w3491:string, time string=w3488:string)  [unwired: 2 in]
                    n2470 = local read "Remarks :"() -> (w3467:string)
                    n2471 = Concatenate Strings("Load :- " ("Substring"), w3480, " grams ," ("Substring")) -> (w3479:string)
                    n2472 = local read "String 41"() -> (w3459:string)
                    n2473 = Concatenate Strings(w3468) -> (w3469:string)
                    n2474 = Concatenate Strings(w3456) -> (w3455:string)
                    n2475 = Concatenate Strings("tested by") -> (w3463:string)
                    n2476 = Concatenate Strings("(" ("Substring"), w3491, ")" ("Substring"), w3488) -> (w3461:string)
                    "concatenated string" <- w3461
                    n2477 = Concatenate Strings(w3467, "," ("string")) -> (w3466:string)
                    n2478 = Concatenate Strings("  TIME;      COF;       STROKE;     AIR TEMP;  TEMP;  HUMIDITY;  ECR; PID-OUT; FREQUENCY" ("Substring"), "\r") -> (w3475:string)
                    n2479 = Concatenate Strings(w3459, w3458, "Fuel Discription :-" ("Substring"), w3469, w3458, w3479, w3458, "Batch Ref Num :-" ("Substring"), w3455, w3458, " Remarks :- " ("Substring"), w3466, w3458, " Date :- " ("Substring"), w3461, w3458, "Tested By :-" ("Substring"), w3463) -> (w3473:string)
                    "REMARKS" <- w3473
                    n2480 = call <vilib>:"Write Characters To File.vi"("append to file? (new file:F)"=FALSE, "character string"=w3475, "file path (dialog if empty)"=w3443) -> ()  [unwired: 2 in, 1 out]
                    n2481 = call <vilib>:"Write Characters To File.vi"("append to file? (new file:F)"=FALSE, "character string"=w3473, "file path (dialog if empty)"=w3442) -> ()  [unwired: 2 in, 1 out]
                  }
                  frame #2 {
                    n2482 = local write "Cycles elapsed"(0 ("Cycles elapsed")) -> ()
                    n2483 = local write "cyclecount"(0 ("cyclecount")) -> ()
                    n2484 = local write "Save & Continue"(FALSE ("OK")) -> ()
                    n2485 = local write "autostrtflg"(TRUE ("autostrtflg")) -> ()
                    n2486 = local write "Save"(FALSE ("Save")) -> ()
                    n2487 = Get Date/Time In Seconds() -> (seconds since 1Jan1904=w3498:timestamp)
                    n2488 = To Double Precision Float(number=w3498) -> (double precision float=w3497:dbl)
                    n2489 = local write "acq timer"(w3497) -> ()
                    n2490 = One Button Dialog(message="Please ensure sample is mounted properly and machine is ready in all aspects for testing !", button name ("OK")="Ok") -> ()  [unwired: 1 out]
                  }
                  frame #3 {
                    n2491 = stacked-sequence {
                      frame #0 {
                        n2492 = local write "Main Dashboard Buttons"(T1."Dashboard" ("Main Dashboard Buttons")) -> ()
                        n2493 = local write "Main Tab"(T2."Acquire" ("Main Tab")) -> ()
                      }
                      frame #1 {
                        n2494 = local write "EVENT LOG"("" ("EVENT LOG")) -> ()
                      }
                      frame #2 {
                        n2495 = Wait (ms)(milliseconds to wait=u32 50) -> ()  [unwired: 1 out]
                      }
                      frame #3 {
                        n2496 = disable-structure shown="Disabled" {
                          frame Disabled {
                            n2497 = local read "EVENT LOG"() -> (w3510:string)
                            n2498 = call "Event Log.vi"("Content"="Test Details", "EVENT LOG"=w3510) -> ("EVENT LOG"=w3509:string)  [unwired: 8 in, 1 out]
                            n2499 = local write "EVENT LOG"(w3509) -> ()
                          }
                          frame Enabled {
                          }
                        }
                      }
                      frame #4 {
                        n2500 = Wait (ms)(milliseconds to wait=u32 50) -> ()  [unwired: 1 out]
                      }
                      frame #5 {
                        n2501 = local read "FILE"() -> (w3512:string)
                        n2502 = Concatenate Strings("File Name :" ("Content"), w3512) -> (w3513:string)
                        n2503 = local read "EVENT LOG"() -> (w3516:string)
                        n2504 = call "Event Log.vi"("Content"=w3513, "EVENT LOG"=w3516) -> ("EVENT LOG"=w3515:string)  [unwired: 8 in, 1 out]
                        n2505 = local write "EVENT LOG"(w3515) -> ()
                      }
                      frame #6 {
                        n2506 = Wait (ms)(milliseconds to wait=u32 50) -> ()  [unwired: 1 out]
                      }
                      frame #7 {
                        n2507 = local read "Batch Ref Num :"() -> (w3518:string)
                        n2508 = Concatenate Strings("Batch Ref No :" ("Content"), w3518) -> (w3519:string)
                        n2509 = local read "EVENT LOG"() -> (w3522:string)
                        n2510 = call "Event Log.vi"("Content"=w3519, "EVENT LOG"=w3522) -> ("EVENT LOG"=w3521:string)  [unwired: 8 in, 1 out]
                        n2511 = local write "EVENT LOG"(w3521) -> ()
                      }
                      frame #8 {
                        n2512 = Wait (ms)(milliseconds to wait=u32 50) -> ()  [unwired: 1 out]
                      }
                      frame #9 {
                        n2513 = local read "tested by"() -> (w3524:string)
                        n2514 = Concatenate Strings("Tested By :" ("Content"), w3524) -> (w3525:string)
                        n2515 = local read "EVENT LOG"() -> (w3528:string)
                        n2516 = call "Event Log.vi"("Content"=w3525, "EVENT LOG"=w3528) -> ("EVENT LOG"=w3527:string)  [unwired: 8 in, 1 out]
                        n2517 = local write "EVENT LOG"(w3527) -> ()
                      }
                      frame #10 {
                        n2518 = Wait (ms)(milliseconds to wait=u32 50) -> ()  [unwired: 1 out]
                      }
                      frame #11 {
                        n2519 = local read "TEST STANDARD"() -> (w3531:T3)
                        n2520 = case shown="\"ASTM D6079\", Default" w3531 {
                          tunnel: ["ASTM D6079" "ISO 12156" "CEC F-096-A-06" "Custom"] -> w3530
                          frame "ASTM D6079", Default {
                          }
                          frame "ISO 12156" {
                          }
                          frame "CEC F-096-A-06" {
                          }
                          frame "Custom" {
                          }
                        }
                        n2521 = Concatenate Strings("Test Standard :" ("Content"), w3530) -> (w3532:string)
                        n2522 = local read "EVENT LOG"() -> (w3535:string)
                        n2523 = call "Event Log.vi"("Content"=w3532, "EVENT LOG"=w3535) -> ("EVENT LOG"=w3534:string)  [unwired: 8 in, 1 out]
                        n2524 = local write "EVENT LOG"(w3534) -> ()
                      }
                      frame #12 {
                        n2525 = Wait (ms)(milliseconds to wait=u32 50) -> ()  [unwired: 1 out]
                      }
                      frame #13 {
                        n2526 = local read "Fuel Discription :"() -> (w3541:string)
                        n2527 = Concatenate Strings("Fuel Description :" ("Content"), w3541) -> (w3542:string)
                        n2528 = local read "EVENT LOG"() -> (w3545:string)
                        n2529 = call "Event Log.vi"("Content"=w3542, "EVENT LOG"=w3545) -> ("EVENT LOG"=w3544:string)  [unwired: 8 in, 1 out]
                        n2530 = local write "EVENT LOG"(w3544) -> ()
                      }
                      frame #14 {
                        n2531 = Wait (ms)(milliseconds to wait=u32 50) -> ()  [unwired: 1 out]
                      }
                      frame #15 {
                        n2532 = local read "Remarks :"() -> (w3547:string)
                        n2533 = Concatenate Strings("Remarks :" ("Content"), w3547) -> (w3548:string)
                        n2534 = local read "EVENT LOG"() -> (w3551:string)
                        n2535 = call "Event Log.vi"("Content"=w3548, "EVENT LOG"=w3551) -> ("EVENT LOG"=w3550:string)  [unwired: 8 in, 1 out]
                        n2536 = local write "EVENT LOG"(w3550) -> ()
                      }
                      frame #16 {
                        n2537 = Wait (ms)(milliseconds to wait=u32 50) -> ()  [unwired: 1 out]
                      }
                      frame #17 {
                        n2538 = local read "Operator ID"() -> (w3553:string)
                        n2539 = Concatenate Strings("Operator ID :" ("Content"), w3553) -> (w3555:string)
                        n2540 = local read "EVENT LOG"() -> (w3557:string)
                        n2541 = call "Event Log.vi"("Content"=w3555, "EVENT LOG"=w3557) -> ("EVENT LOG"=w3556:string)  [unwired: 8 in, 1 out]
                        n2542 = local write "EVENT LOG"(w3556) -> ()
                      }
                      frame #18 {
                        n2543 = Wait (ms)(milliseconds to wait=u32 50) -> ()  [unwired: 1 out]
                      }
                      frame #19 {
                        n2544 = disable-structure shown="Disabled" {
                          frame Disabled {
